vi "AvoidFault.vi"(8 "error in (no error)":errorcluster, 9 "Game":refnum<class "Game.lvclass">, 10 "Robot in":refnum<class "Robot.lvclass">, 11 "MarkerTactic in":refnum<class "MarkerTactic.lvclass">) -> (0 "error out":errorcluster, 2 "Robot out":refnum<class "Robot.lvclass">, 3 "MarkerTactic out":refnum<class "MarkerTactic.lvclass">)   [LabVIEW 2023, in "MarkerTactic.lvclass"]
uses:
  MarkerTactic.lvclass
  Robot_class/Robot.lvclass
  Game_class/Game.lvclass
  Game_class/Game.lvclass/Game.ctl
  Team_class/Team.lvclass/Team.ctl
  Object_class/Object.lvclass/Object.ctl
  Parameters_class/Parameters.lvclass/Parameters.ctl
  Robot_class/Robot.lvclass/Robot.ctl
  Robot_class/Write dest_x.vi
  Robot_class/Write dest_y.vi
  Robot_class/Write dest_orientation.vi
  Object_class/Read x.vi
  Object_class/Read y.vi
  Robot_class/Read dest_x.vi
  Robot_class/Read dest_y.vi
  Game_class/Read Utilities.lvclass.vi
  Game_class/Read OffensiveTeam.vi
  Game_class/Read BallRef.vi
  Game_class/Read Parameters.lvclass.vi
  Parameters_class/Read DistanceStop.vi
  Team_class/Read RobotRef.vi
  Ball_class/Ball.lvclass
  Ally_class/Ally.lvclass
  Utilities_class/Utilities.lvclass
  Parameters_class/Parameters.lvclass
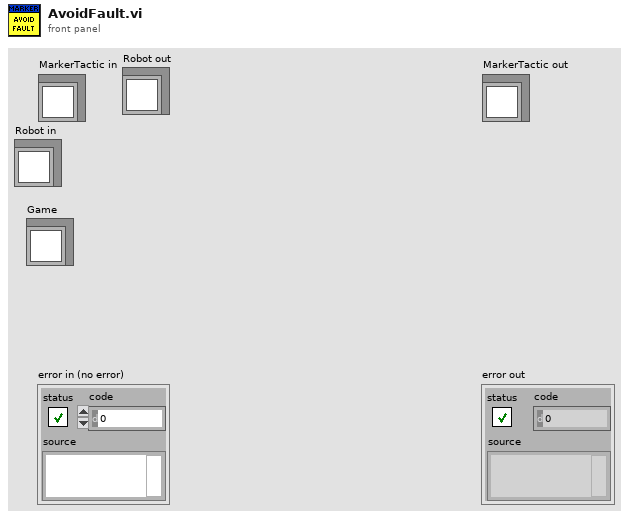
[diagram p1: front panel]
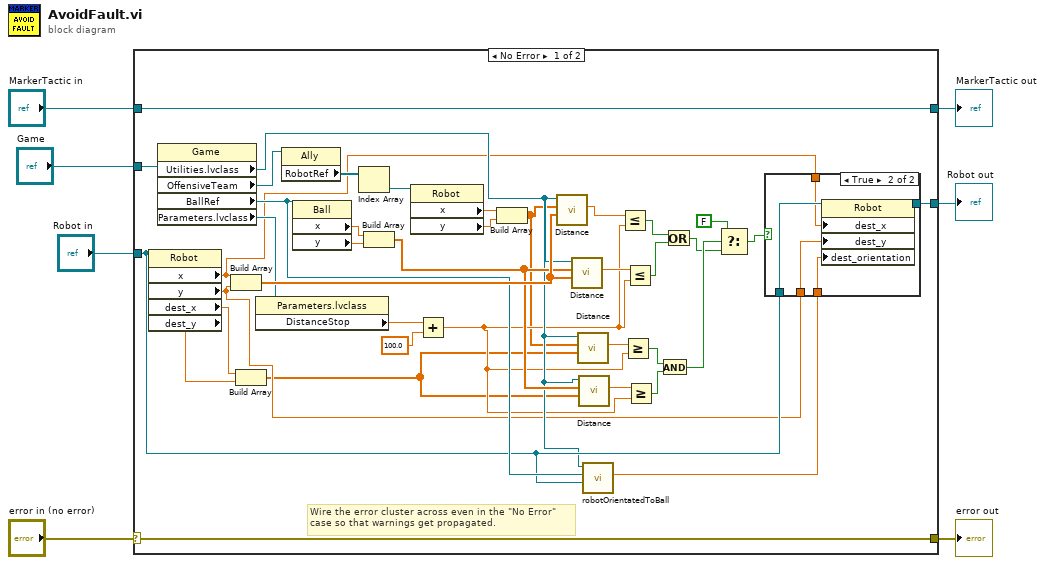
[diagram p0: block diagram]
diagram:
  n1 = case shown="No Error" "error in (no error)" {
    selector: "error in (no error)" -> [w45 w54]
    tunnel: [w45 w54] -> w6
    tunnel: [w46 w53] -> w4
    tunnel: "MarkerTactic in" -> [w46 w53]
    tunnel: "Game" -> [w44 _]
    tunnel: "Robot in" -> [w25 _]
    tunnel: [w30 _] -> w1
    frame No Error {
      # "Wire the error cluster across even in the \"No Error\"\ncase so that warnings get propagated."
      n2 = property class="Robot"(reference=w25) -> ("x"=w11:dbl, "y"=w10:dbl, "dest_x"=w24:dbl, "dest_y"=w23:dbl)  [unwired: 1 in, 2 out]
      n3 = property class="Game"(reference=w44) -> ("Utilities.lvclass"=w21:refnum<class "Utilities.lvclass">, "OffensiveTeam"=w43:refnum<class "Ally.lvclass">, "BallRef"=w26:refnum<class "Ball.lvclass">, "Parameters.lvclass"=w34:refnum<class "Parameters.lvclass">)  [unwired: 1 in, 2 out]
      n4 = Build Array(w11, w10) -> (w36:dbl[])
      n5 = Build Array(w24, w23) -> (w8:dbl[])
      n6 = property class="Parameters.lvclass"(reference=w34) -> ("DistanceStop"=w29:dbl)  [unwired: 1 in, 2 out]
      n7 = property class="Ally"(reference=w43) -> ("RobotRef"=w42:refnum<class "Robot.lvclass">[])  [unwired: 1 in, 2 out]
      n8 = property class="Ball"(reference=w26) -> ("x"=w40:dbl, "y"=w39:dbl)  [unwired: 1 in, 2 out]
      n9 = Index Array(array=w42) -> (element=w41:refnum<class "Robot.lvclass">)  [unwired: 1 in]
      n10 = Build Array(w40, w39) -> (w22:dbl[])
      n11 = property class="Robot"(reference=w41) -> ("x"=w38:dbl, "y"=w37:dbl)  [unwired: 1 in, 2 out]
      n12 = Add(x=w29, y=100.0) -> (x+y=w18:dbl)
      n13 = Build Array(w38, w37) -> (w9:dbl[])
      n14 = call-dynamic "Distance.vi"("P1"=w36, "P2"=w9, "Utilities in"=w21) -> ("Distance"=w35:dbl)  [unwired: 6 in, 2 out]
      n15 = call-dynamic "Distance.vi"("P1"=w36, "P2"=w22, "Utilities in"=w21) -> ("Distance"=w33:dbl)  [unwired: 6 in, 2 out]
      n16 = call-dynamic "Distance.vi"("P1"=w8, "P2"=w9, "Utilities in"=w21) -> ("Distance"=w20:dbl)  [unwired: 6 in, 2 out]
      n17 = call-dynamic "Distance.vi"("P1"=w8, "P2"=w22, "Utilities in"=w21) -> ("Distance"=w19:dbl)  [unwired: 6 in, 2 out]
      n18 = call "robotOrientatedToBall.vi"("Robot"=w25, "BallRef"=w26, "Utilities in"=w21) -> ("Orientation"=w27:dbl)  [unwired: 6 in, 2 out]
      n19 = Less Or Equal?(x=w35, y=w18) -> (x <= y?=w32:bool)
      n20 = Greater Or Equal?(x=w20, y=w18) -> (x >= y?=w17:bool)
      n21 = Less Or Equal?(x=w33, y=w18) -> (x <= y?=w31:bool)
      n22 = Greater Or Equal?(x=w19, y=w18) -> (x >= y?=w16:bool)
      n23 = And(x=w17, y=w16) -> (x .and. y?=w15:bool)
      n24 = Or(x=w32, y=w31) -> (x .or. y?=w13:bool)
      n25 = Select(t=FALSE, s=w15, f=w13) -> (s? t:f=w12:bool)
      n26 = case shown="True" w12 {
        tunnel: [w47 w52] -> w30
        tunnel: w25 -> [w47 w51]
        tunnel: w27 -> [_ w50]
        tunnel: w11 -> [_ w49]
        tunnel: w10 -> [_ w48]
        frame False {
        }
        frame True {
          n27 = property class="Robot"(reference=w51, "dest_x"=w49, "dest_y"=w48, "dest_orientation"=w50) -> (reference out=w52:refnum<class "Robot.lvclass">)  [unwired: 1 in, 1 out]
        }
      }
    }
    frame Error {
    }
  }
  "error out" <- w6
  "MarkerTactic out" <- w4
  "Robot out" <- w1
